vi "Running Average with Shift Registers.vi"() -> ()   [LabVIEW 2023]
doc: "Uses a While Loop with shift registers to calculate the 4-point running average of random data. A Waveform Chart displays both the raw and averaged data."
panel:
  in  "Stop":bool
  out "Random Plot":cluster{dbl, dbl}(graph)
  # "Overview: Demonstrates the use of Shift Registers to calculate a running average.\nInstructions:\n1. Run the VI. The Random Plot will display the current random value, and a running average of the four most recent values.\n2. Click Stop to stop the VI."
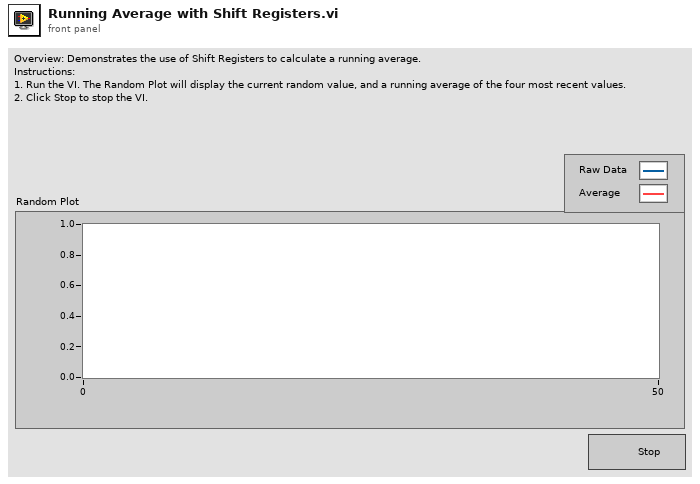
[diagram p1: front panel]
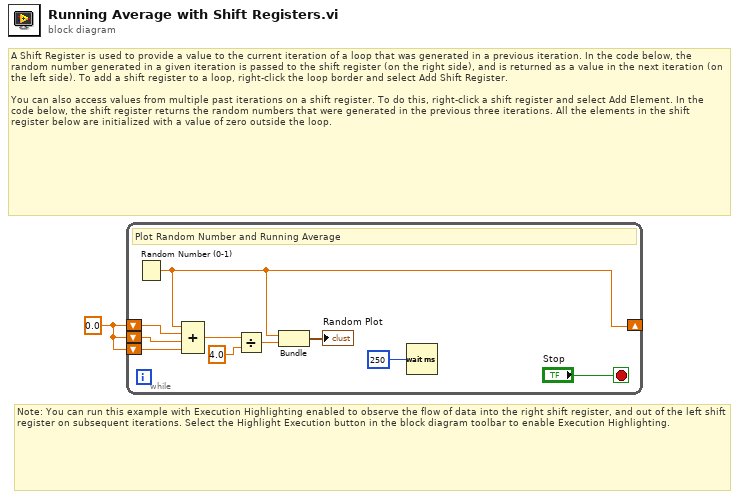
[diagram p0: block diagram]
diagram:
  w1 = 0.0
  # "Note: You can run this example with Execution Highlighting enabled to observe the flow of data into the right shift register, and out of the left shift register on subsequent iterations. Select the Highlight Execution button in the block diagram toolbar to enable Execution Highlighting."
  # "A Shift Register is used to provide a value to the current iteration of a loop that was generated in a previous iteration. In the code below, the random number generated in a given iteration is passed to the shift register (on the right side), and is returned as a value in the next iteration (on the left side). To add a shift register to a loop, right-click the loop border and select Add Shift Register.\n\nYou can also access values from multiple past iterations on a shift register. To do this, right-click a shift register and select Add Element. In the code below, the shift register returns the random numbers that were generated in the previous three iterations. All the elements in the shift register below are initialized with a value of zero outside the loop."
  n1 = while {
    shift-left: w1 -> [w7]
    shift-left: w1 -> [w6]
    shift-left: w1 -> [w5]
    shift-right: [w4] -> _
    stop <- "Stop" stop-if-true
    # "Plot Random Number and Running Average"
    n2 = Random Number (0-1)() -> (number: 0 to 1=w4:dbl)
    n3 = Compound Arithmetic op=ADD(w4, w5, w6, w7) -> (w3:dbl)
    n4 = Divide(x=w3, y=4.0) -> (x/y=w10:dbl)
    n5 = Bundle(w4, w10) -> (→"Random Plot":cluster{dbl, dbl})  [unwired: 1 in]
    n6 = Wait (ms)(milliseconds to wait=u32 250) -> ()  [unwired: 1 out]
  }
